vi "Config.vi"(8 "error in (no error)":errorcluster, 10 "JSON config":string, 11 "MQTTclient in":refnum<class "MQTTclient.lvclass">) -> (0 "error out":errorcluster, 3 "MQTTclient out":refnum<class "MQTTclient.lvclass">)   [LabVIEW 2015, in "MQTTclient.lvclass"]
uses:
  MQTTclient.lvclass
  config.ctl
  MQTTclient.lvclass/MQTTclient.ctl
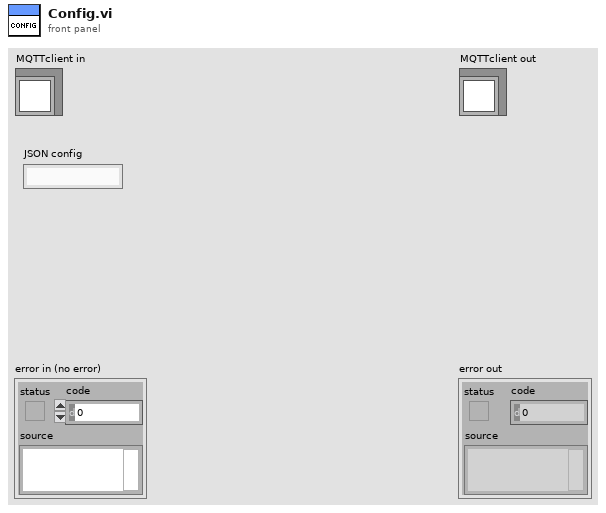
[diagram p1: front panel]
types:
  T1 = typedef "MQTTclient.lvclass/config.ctl" = cluster{"Broker":cluster{"IP":string, "port":u16, "connTimeout":i32, "writeTimeout":i32, "readTimeout":i32, "subTimeout":i32}, "Connect Flags":cluster{"reserved":bool, "clean session":bool, "will flag":bool, "willQOS":string, "will retain":bool, "password":bool, "user name":bool}, "Keep Alive":u16, "Client Info":cluster{"ClientId":string, "Will Topic":string, "Will Message":string, "User Name":string, "Password":string}}
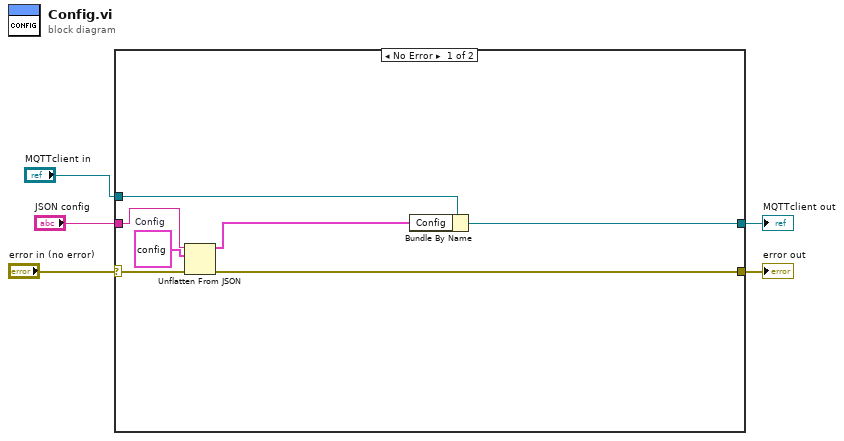
[diagram p0: block diagram]
diagram:
  n1 = case shown="No Error" "error in (no error)" {
    selector: "error in (no error)" -> [w7 w14]
    tunnel: [w8 w14] -> w4
    tunnel: [w10 w13] -> w2
    tunnel: "MQTTclient in" -> [w6 w13]
    tunnel: "JSON config" -> [w12 _]
    frame No Error {
      w11 = T1 {"Broker"={"IP"="", "port"=0, "connTimeout"=0, "writeTimeout"=0, "readTimeout"=0, "subTimeout"=0}, "Connect Flags"={"reserved"=FALSE, "clean session"=FALSE, "will flag"=FALSE, "willQOS"="", "will retain"=FALSE, "password"=FALSE, "user name"=FALSE}, "Keep Alive"=0, "Client Info"={"ClientId"="", "Will Topic"="", "Will Message"="", "User Name"="", "Password"=""}}  # Config
      n2 = Unflatten From JSON(JSON string=w12, type and defaults=w11, error in (no error)=w7) -> (value=w9:T1, error out=w8:errorcluster)  [unwired: 4 in]
      n3 = Bundle By Name(cluster=w6, "Config"=w9) -> (w10:refnum<class "MQTTclient.lvclass">)
    }
    frame Error {
    }
  }
  "error out" <- w4
  "MQTTclient out" <- w2
